vi "Acquire.vi"(8 "error in (no error)":errorcluster, 10 "Capacitive Readout Notifier":refnum<notifier>, 11 "Hardware Refs In":T1={"IP Address"="Simulator", "Handle"=0, "Refresh Time (ms)"=0.0}) -> (0 "error out":errorcluster, 3 "Hardware Refs Out":T1={"IP Address"="Simulator", "Handle"=0, "Refresh Time (ms)"=0.0})   [LabVIEW 2013, in "Capacitive.lvlib"]
uses:
  Capacitive.lvlib
  Hardware Configuration.ctl
  Piezo/Piezo display.ctl
  Capacitive Signal Cluster.ctl
  Desktop/Simon Labview/Piezo.lvlib
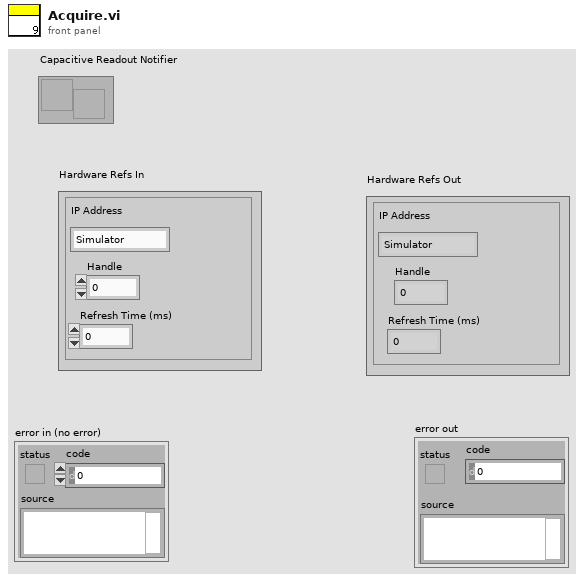
[diagram p1: front panel]
types:
  T1 = typedef "Capacitive.lvlib/Hardware Configuration.ctl" = cluster{"IP Address":string, "Handle":u32, "Refresh Time (ms)":dbl}
  T2 = typedef "Capacitive.lvlib/Capacitive Signal Cluster.ctl" = cluster{"Readout":sgl, "Time":i32}
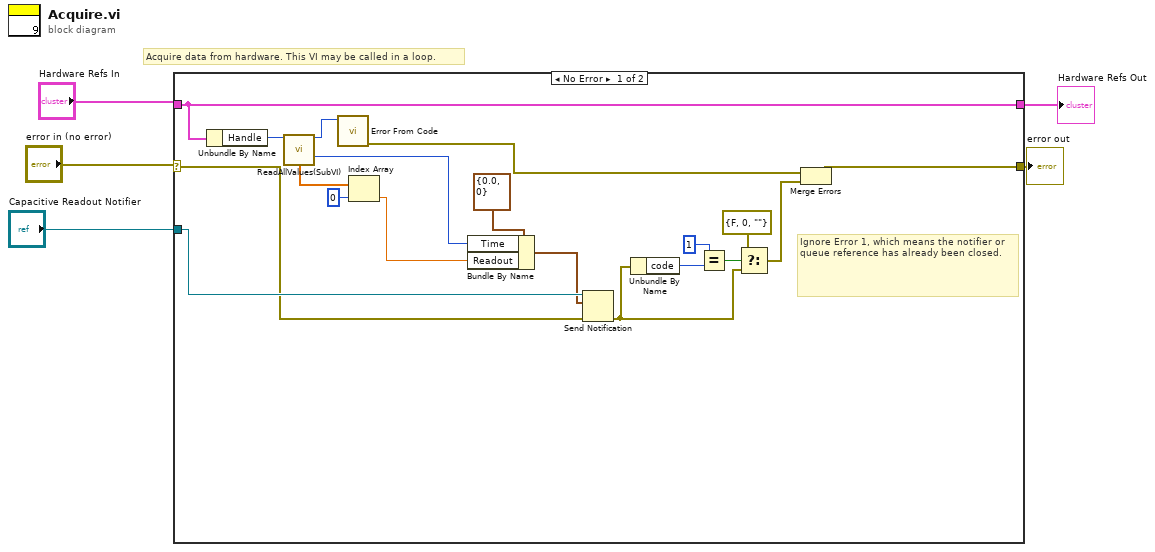
[diagram p0: block diagram]
diagram:
  # "Acquire data from hardware. This VI may be called in a loop."
  n1 = case shown="No Error" "error in (no error)" {
    selector: "error in (no error)" -> [w8 w25]
    tunnel: [w24 w25] -> w4
    tunnel: "Hardware Refs In" -> [w14 w26]
    tunnel: [w14 w26] -> w3
    tunnel: "Capacitive Readout Notifier" -> [w18 _]
    frame No Error {
      # "Ignore Error 1, which means the notifier or queue reference has already been closed."
      n2 = Unbundle By Name(w14) -> ("Handle"=w13:u32)
      n3 = call "ReadAllValues(SubVI).vi"("Handle in"=w13) -> ("Status"=w7:i32, "Timestamp"=w9:u64, "Displacement"=w12:dbl[])  [unwired: 8 in, 4 out]
      n4 = call "Error From Code.vi"("ErrorCode"=w7) -> ("error out"=w6:errorcluster)  [unwired: 10 in]
      n5 = Index Array(array=w12, index=0) -> (element=w10:dbl)
      n6 = Bundle By Name(cluster=T2 {"Readout"=0.0, "Time"=0} ("Capacitive Signal Cluster"), "Time"=w9, "Readout"=w10) -> (w16:T2)
      n7 = Send Notification(notification=w16, notifier=w18, error in (no error)=w8) -> (error out=w17:errorcluster)  [unwired: 1 out]
      n8 = Unbundle By Name(w17) -> ("code"=w23:i32)
      n9 = Equal?(x=1, y=w23) -> (x = y?=w21:bool)
      n10 = Select(t=errorcluster {"status"=FALSE, "code"=0, "source"=""} ("error constant"), s=w21, f=w17) -> (s? t:f=w20:errorcluster)
      n11 = Merge Errors(w6, w20) -> (w24:errorcluster)
    }
    frame Error {
    }
  }
  "error out" <- w4
  "Hardware Refs Out" <- w3
